vi "H5Pget_filter.vi"(8 "error in (no error)":errorcluster, 10 "Filter Index":u32, 11 "HDF5 Property Ref":T3) -> (0 "error out":errorcluster, 1 "Filter Name":string, 2 "Filter":T2 items=["H5Z_FILTER_ERROR"=-1, "H5Z_FILTER_NONE"=0, "H5Z_FILTER_DEFLATE"=1, "H5Z_FILTER_SHUFFLE"=2, "H5Z_FILTER_FLETCHER32"=3, "H5Z_FILTER_SZIP"=4], 3 "HDF5 Ref out":T3, 4 "cd_values":u32[](array[numeric]), 5 "Filter Flag":T1 items=["H5Z_FLAG_MANDATORY"=0, "H5Z_FLAG_OPTIONAL"=1, "H5Z_FLAG_REVERSE"=256, "H5Z_FLAG_SKIP_EDC"=512], 7 "Filter Config":u32)   [LabVIEW 2017]
doc: "Returns information about a filter in a pipeline.\n <p>"
uses:
  <vilib>/UPVI/lvhdf5/library.llb/HDF5 Ref.ctl
  <vilib>/UPVI/lvhdf5/property.llb/H5Z_filter_t.ctl
  <vilib>/UPVI/lvhdf5/property.llb/H5Z_flag_t.ctl
  <vilib>/UPVI/lvhdf5/hdf5.dll
panel:
  # "LVHDF5 Toolkit\nCopyright (c) 2005-2013 by Jason D. Sommerville\nCopyright (c) 2014 by UPVI, LLC.\n\nThis use and distribution of this file is governed by the terms found in \nLICENSE.txt distributed with this toolkit and installed at\n <user.lib>\\_lvhdf5\\LICENSE.txt"
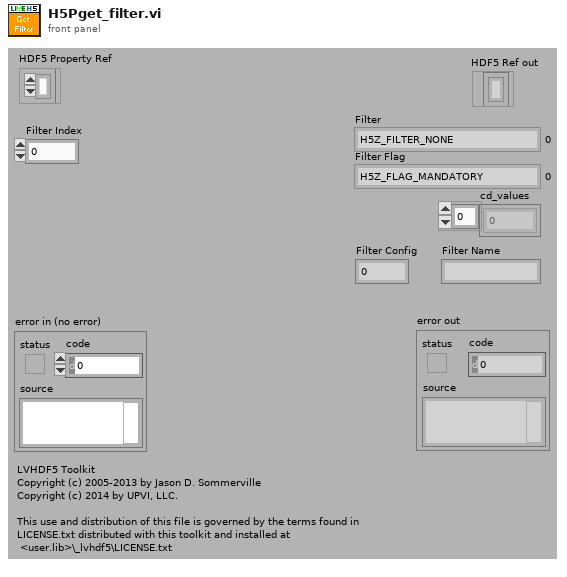
[diagram p1: front panel]
types:
  T1 = typedef "H5Z_flag_t.ctl" = u32
  T2 = typedef "H5Z_filter_t.ctl" = i32
  T3 = typedef "HDF5 Ref.ctl" = refnum<k1>
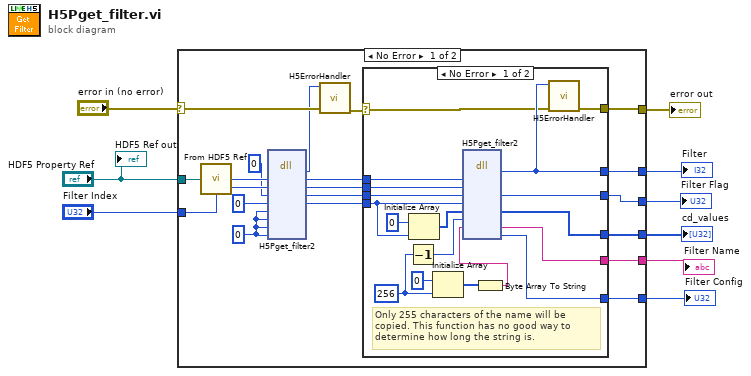
[diagram p0: block diagram]
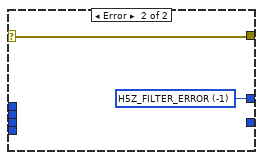
[diagram p2: hidden frame]
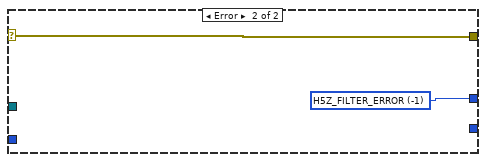
[diagram p3: hidden frame]
diagram:
  n1 = case shown="No Error" "error in (no error)" {
    selector: "error in (no error)" -> [w16 w50]
    tunnel: [w28 w50] -> w8
    tunnel: "HDF5 Property Ref" -> [w27 _]
    tunnel: [w26 w49] -> w6
    tunnel: "Filter Index" -> [w20 _]
    tunnel: [w25 _] -> w4
    tunnel: [w13 _] -> w3
    tunnel: [w12 _] -> w2
    tunnel: [w10 _] -> w1
    frame No Error {
      w11 = u32 0 ("namelen")
      n2 = call <vilib>:"From HDF5 Ref.vi"("HDF5 Ref"=w27) -> ("I32"=w21:i32)
      n3 = dll-call lib="C:/Program Files/National Instruments/LabVIEW 2017/vi.lib/UPVI/lvhdf5/hdf5.dll" fn="H5Pget_filter2" label="H5Pget_filter"("plist_id"=w21, "filter_number"=w20, "flags"=u32 0, "cd_nelmts"=u32 0, "cd_values"=w11, "namelen"=w11, "name"=w11, "filter_config"=w11) -> ("return type"=w15:i32, "plist_id"=w22:i32, "filter_number"=w23:u32, "flags"=w18:u32, "cd_nelmts"=w17:u64)  [unwired: 7 in, 2 out]
      n4 = call <vilib>:"H5ErrorHandler.vi"("error in (no error)"=w16, "herr_t"=w15) -> ("error out"=w14:errorcluster)  [unwired: 3 in, 4 out]
      n5 = case shown="No Error" w14 {
        selector: w14 -> [w40 w47]
        tunnel: [w46 w47] -> w28
        tunnel: [w45 w48] -> w26
        tunnel: w23 -> [w44 _]
        tunnel: [w43 _] -> w25
        tunnel: w22 -> [w42 _]
        tunnel: w18 -> [w41 _]
        tunnel: w17 -> [w37 _]
        tunnel: [w31 _] -> w13
        tunnel: [w30 _] -> w12
        tunnel: [w29 _] -> w10
        frame No Error {
          w35 = 256 ("dimension size")
          # "Only 255 characters of the name will be copied. This function has no good way to determine how long the string is."
          n6 = Decrement(x=w35) -> (x-1=w34:i32)
          n7 = Initialize Array(u32 0, w37) -> (w38:u32[])
          n8 = Initialize Array(u8 0 ("element"), w35) -> (w33:u8[])
          n9 = Byte Array To String(unsigned byte array=w33) -> (string=w32:string)
          n10 = dll-call lib="C:/Program Files/National Instruments/LabVIEW 2017/vi.lib/UPVI/lvhdf5/hdf5.dll" fn="H5Pget_filter2" label="H5Pget_filter"("plist_id"=w42, "filter_number"=w44, "flags"=w41, "cd_nelmts"=w37, "cd_values"=w38, "namelen"=w34, "name"=w32) -> ("return type"=w45:i32, "flags"=w43:u32, "cd_values"=w31:u32[], "name"=w30:string, "filter_config"=w29:u32)  [unwired: 8 in, 2 out]
          n11 = call <vilib>:"H5ErrorHandler.vi"("error in (no error)"=w40, "herr_t"=w45) -> ("error out"=w46:errorcluster)  [unwired: 3 in, 4 out]
        }
        frame Error {
          w48 = T2 -1 items=["H5Z_FILTER_ERROR"=-1, "H5Z_FILTER_NONE"=0, "H5Z_FILTER_DEFLATE"=1, "H5Z_FILTER_SHUFFLE"=2, "H5Z_FILTER_FLETCHER32"=3, "H5Z_FILTER_SZIP"=4] ("Filter")
        }
      }
    }
    frame Error {
      w49 = T2 -1 items=["H5Z_FILTER_ERROR"=-1, "H5Z_FILTER_NONE"=0, "H5Z_FILTER_DEFLATE"=1, "H5Z_FILTER_SHUFFLE"=2, "H5Z_FILTER_FLETCHER32"=3, "H5Z_FILTER_SZIP"=4] ("Filter")
    }
  }
  "error out" <- w8
  "Filter" <- w6
  "Filter Flag" <- w4
  "cd_values" <- w3
  "Filter Name" <- w2
  "Filter Config" <- w1
  "HDF5 Ref out" <- "HDF5 Property Ref"
